vi "ACT target_value_matching_value.vi"(0 "MD420.lvclass":refnum<class "MD420.lvclass">, 1 "PG eff SP":dbl, 2 "PG 2nd Min in %":dbl, 3 "PG target SP":dbl, 4 "PUMA RELEB GW81":bool, 5 "ACT 2nd Ctrl":dbl, 6 "ACT limit Setpoint":dbl, 7 "error in (no error)":errorcluster) -> (20 "MD420.lvclass out":refnum<class "MD420.lvclass">, 22 "PG Eff SP":dbl, 24 "Internal Outputs":T1, 27 "error out":errorcluster)   [LabVIEW 2022 SP3, in "MD420.lvclass"]
uses:
  MD420.lvclass
  MD420.lvclass/MD420.ctl
panel:
  # "MD420"
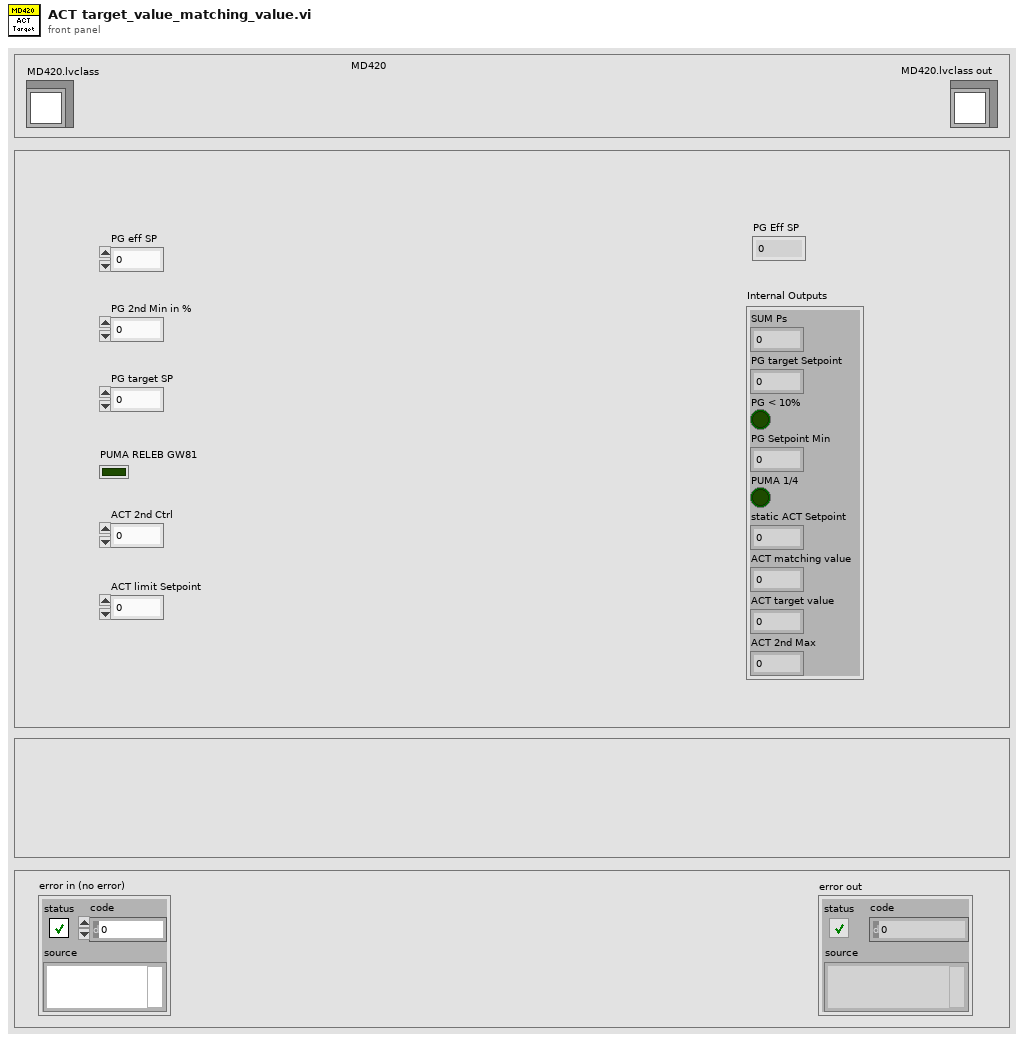
[diagram p1: front panel]
types:
  T1 = cluster{"SUM Ps":dbl, "PG target Setpoint":dbl, "PG < 10%":bool, "PG Setpoint Min":dbl, "PUMA 1/4":bool, "static ACT Setpoint":dbl, "ACT matching value":dbl, "ACT target value":dbl, "ACT 2nd Max":dbl}
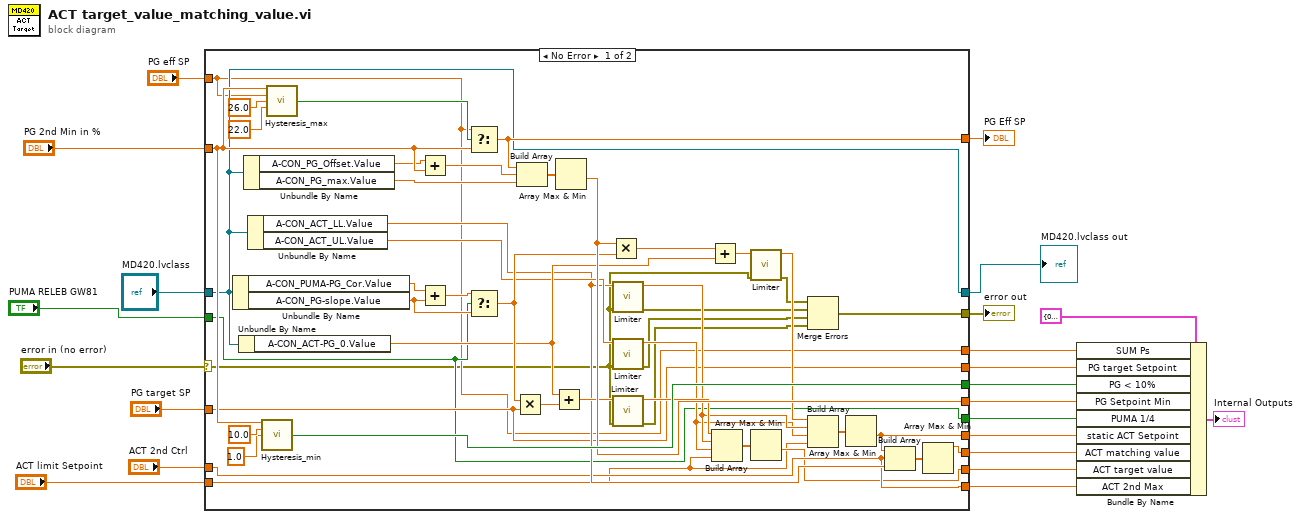
[diagram p0: block diagram]
diagram:
  n1 = case shown="No Error" "error in (no error)" {
    selector: "error in (no error)" -> [w28 w70]
    tunnel: [w23 w70] -> w21
    tunnel: "MD420.lvclass" -> [w34 w69]
    tunnel: [w34 w69] -> w19
    tunnel: "PG eff SP" -> [w31 _]
    tunnel: "PG 2nd Min in %" -> [w62 _]
    tunnel: "PG target SP" -> [w33 _]
    tunnel: "PUMA RELEB GW81" -> [w32 _]
    tunnel: "ACT 2nd Ctrl" -> [w37 _]
    tunnel: [w60 _] -> w3
    tunnel: [w63 _] -> w10
    tunnel: [w53 _] -> w9
    tunnel: [w38 _] -> w6
    tunnel: [w37 _] -> w4
    tunnel: [w35 _] -> w5
    tunnel: [w33 _] -> w11
    tunnel: [w32 _] -> w8
    tunnel: [w31 _] -> w12
    tunnel: "ACT limit Setpoint" -> [w30 _]
    tunnel: [w29 _] -> w7
    frame No Error {
      n2 = Unbundle By Name(w34) -> ("A-CON_PUMA-PG_Cor.Value"=w56:dbl, "A-CON_PG-slope.Value"=w54:dbl)
      n3 = Unbundle By Name(w34) -> ("A-CON_ACT-PG_0.Value"=w49:dbl)
      n4 = Unbundle By Name(w34) -> ("A-CON_PG_Offset.Value"=w61:dbl, "A-CON_PG_max.Value"=w58:dbl)
      n5 = Unbundle By Name(w34) -> ("A-CON_ACT_LL.Value"=w40:dbl, "A-CON_ACT_UL.Value"=w46:dbl)
      n6 = call "Hysteresis_min.vi"("input"=w62, "Min"=10.0, "H"=1.0) -> ("Deviation"=w63:bool)  [unwired: 11 in, 1 out]
      n7 = call "Hysteresis_max.vi"("input(+)"=w62, "input (-)"=w31, "H"=26.0 ("Min"), "Max"=22.0 ("H")) -> ("Deviation"=w68:bool)  [unwired: 10 in, 1 out]
      n8 = Add(x=w61, y=w62) -> (x+y=w59:dbl)
      n9 = Add(x=w56, y=w54) -> (x+y=w55:dbl)
      n10 = Select(t=w31, s=w68, f=w62) -> (s? t:f=w60:dbl)
      n11 = Select(t=w55, s=w32, f=w54) -> (s? t:f=w52:dbl)
      n12 = Multiply(x=w52, y=w33) -> (x*y=w50:dbl)
      n13 = Build Array(w60, w59, w58) -> (w57:dbl[])
      n14 = Add(x=w49, y=w50) -> (x+y=w47:dbl)
      n15 = Array Max & Min(array=w57) -> (min value=w53:dbl)  [unwired: 3 out]
      n16 = Multiply(x=w53, y=w52) -> (x*y=w51:dbl)
      n17 = call "Limiter.vi"("error in"=w28, "input"=w40) -> ("error IO"=w26:errorcluster, "LIMITER_PG_lift-up.UL out"=w43:dbl)  [unwired: 6 in, 2 out]
      n18 = call "Limiter.vi"("error in"=w28, "input"=w46) -> ("error IO"=w25:errorcluster, "LIMITER_PG_lift-up.UL out"=w42:dbl)  [unwired: 6 in, 2 out]
      n19 = call "Limiter.vi"("error in"=w28, "input"=w47) -> ("error IO"=w24:errorcluster, "LIMITER_PG_lift-up.UL out"=w44:dbl)  [unwired: 6 in, 2 out]
      n20 = Add(x=w51, y=w49) -> (x+y=w48:dbl)
      n21 = Build Array(w44, w43, w42, w30) -> (w36:dbl[])
      n22 = call "Limiter.vi"("error in"=w28, "input"=w48) -> ("error IO"=w27:errorcluster, "LIMITER_PG_lift-up.UL out"=w45:dbl)  [unwired: 6 in, 2 out]
      n23 = Array Max & Min(array=w36) -> (min value=w35:dbl)  [unwired: 3 out]
      n24 = Merge Errors(w27, w26, w25, w24) -> (w23:errorcluster)
      n25 = Build Array(w45, w43, w42, w30) -> (w41:dbl[])
      n26 = Array Max & Min(array=w41) -> (min value=w29:dbl)  [unwired: 3 out]
      n27 = Build Array(w29, w37, w40) -> (w39:dbl[])
      n28 = Array Max & Min(array=w39) -> (max value=w38:dbl)  [unwired: 3 out]
    }
    frame Error {
    }
  }
  "error out" <- w21
  "MD420.lvclass out" <- w19
  "PG Eff SP" <- w3
  n29 = Bundle By Name(cluster=T1 {"SUM Ps"=0.0, "PG target Setpoint"=0.0, "PG < 10%"=FALSE, "PG Setpoint Min"=0.0, "PUMA 1/4"=FALSE, "static ACT Setpoint"=0.0, "ACT matching value"=0.0, "ACT target value"=0.0, "ACT 2nd Max"=0.0} ("Internal Outputs"), "SUM Ps"=w12, "PG target Setpoint"=w11, "PG < 10%"=w10, "PG Setpoint Min"=w9, "PUMA 1/4"=w8, "static ACT Setpoint"=w7, "ACT matching value"=w6, "ACT target value"=w5, "ACT 2nd Max"=w4) -> (→"Internal Outputs":T1)
